vi "Insert Test.vi"(4 "Unique ID":string, 6 "Insertion Index":i32=-1, 7 "Parent ID":string, 8 "error in (no error)":errorcluster, 9 "Test":refnum<class "Executioner.lvclass">, 10 "Name":string, 11 "Test Executive Ref":refnum<data-value>) -> (0 "error out":errorcluster, 1 "Replaced?":bool, 3 "Test Executive Ref out":refnum<data-value>, 5 "Unique ID out":string)   [LabVIEW 2019, in "Test Executive.lvlib" / "TestExecutive Ref.lvclass"]
uses:
  <vilib>/gpm_packages/@cs/test-executive/Source/Test Executive/TestExecutive Ref/TestExecutive Ref.lvclass
  <vilib>/gpm_packages/@cs/test-executive/Source/Test Executive/ITestExecutive/ITest Executive.lvclass
  <vilib>/gpm_packages/@cs/test-executive/Source/Test Executive/Executioner/Executioner.lvclass
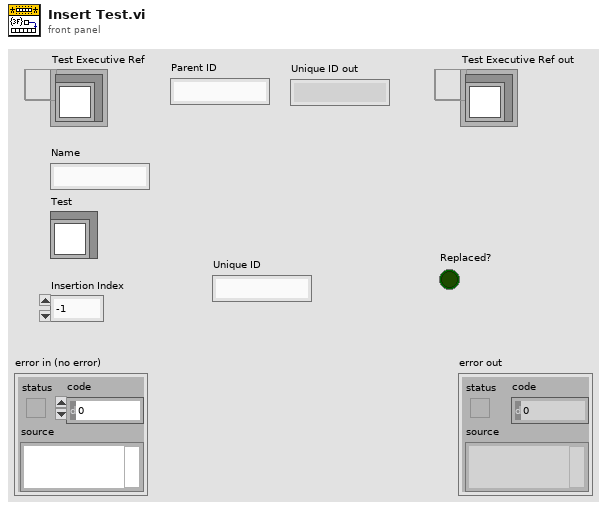
[diagram p1: front panel]
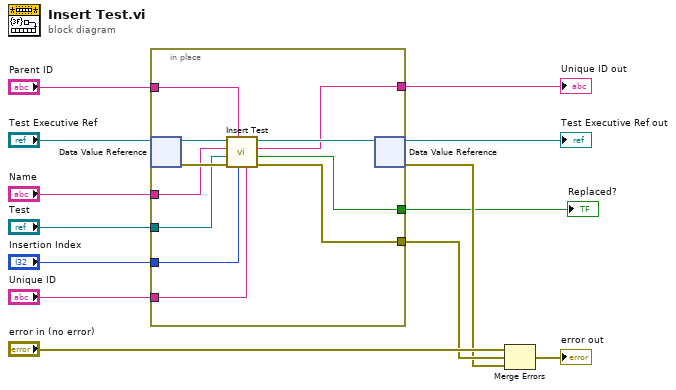
[diagram p0: block diagram]
diagram:
  n1 = in-place {
    in-place-border: "Parent ID" -> [w20]
    in-place-border: [w23] -> w9
    in-place-border: "Name" -> [w19]
    in-place-border: "Test" -> [w18]
    in-place-border: "Insertion Index" -> [w17]
    in-place-border: "Unique ID" -> [w16]
    in-place-border: [w15] -> w2
    in-place-border: [w14] -> w1
    n2 = in-place-dvr #1("Test Executive Ref") -> (w22:refnum<class "ITest Executive.lvclass">, w24:errorcluster)
    n3 = call-dynamic "Insert Test.vi"("Unique ID"=w16, "Insertion Index"=w17, "Parent ID"=w20, "error in (no error)"=w24, "Test"=w18, "Name"=w19, "ITest Executive in"=w22) -> ("error out"=w23:errorcluster, "Replaced?"=w14:bool, "Unique ID out"=w15:string, "ITest Executive out"=w21:refnum<class "ITest Executive.lvclass">)  [unwired: 1 in]
    n4 = in-place-dvr #1(w21) -> (→"Test Executive Ref out":refnum<data-value>, w8:errorcluster)
  }
  "Unique ID out" <- w2
  "Replaced?" <- w1
  n5 = Merge Errors("error in (no error)", w9, w8) -> (→"error out":errorcluster)
